vi "Get Increment.vi"   [LabVIEW 2020, in "Camera.lvclass"]
uses:
  Camera.lvclass
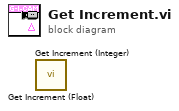
[diagram p0: block diagram]
diagram:
  n1 = call "Get Increment (Float).vi"() -> ()  [unwired: 9 in, 3 out]
  n2 = call "Get Increment (Integer).vi"() -> ()  [unwired: 9 in, 3 out]
